vi "Drive Controller.vi"(8 "error in":errorcluster) -> ()   [LabVIEW 2019]
doc: "This VI executes continuously carrying out the current operation and responding to updates or new operation requests. It will often contain the timing or control code that is difficult to place directly in TeleOp. This VI generally opens all sensors and motors and isolates the rest of the robot code from knowing implementation details of how the operations are carried out."
uses:
  <vilib>/Rock Robotics/WPI/Framework/Completion Status.ctl
  Drive Setpoints.ctl
  Drive Operations.ctl
  <vilib>/Rock Robotics/SystemInterfaces/DIO/FPGA_DIOPWMChannel.ctl
  <vilib>/Rock Robotics/WPI/MotorControl/WPI_MotorControlOpen SPARK.vi
panel:
  in  "Interactive Values":T1
  in  "Buttons":cluster{"Execute Cmd":bool, "Abort Cmd":bool}
  out "Command Timing":cluster{"Start Time (ms)":u32, "Iterations":i32}
  out "Status":T3
  out "Setpoints":T4(graph)
  out "Current\nCmd":string
  # "Tip: The graph shows the motor setpoints. It may also be helpful to observe inputs and sensor values.\nYou may also want to display tuning or debugging controls."
  # "Interactive Command: You may fill in the settings for a command\nand schedule it with the Execute button. You can observe and abort\nany command while fine tuning the code for the controller."
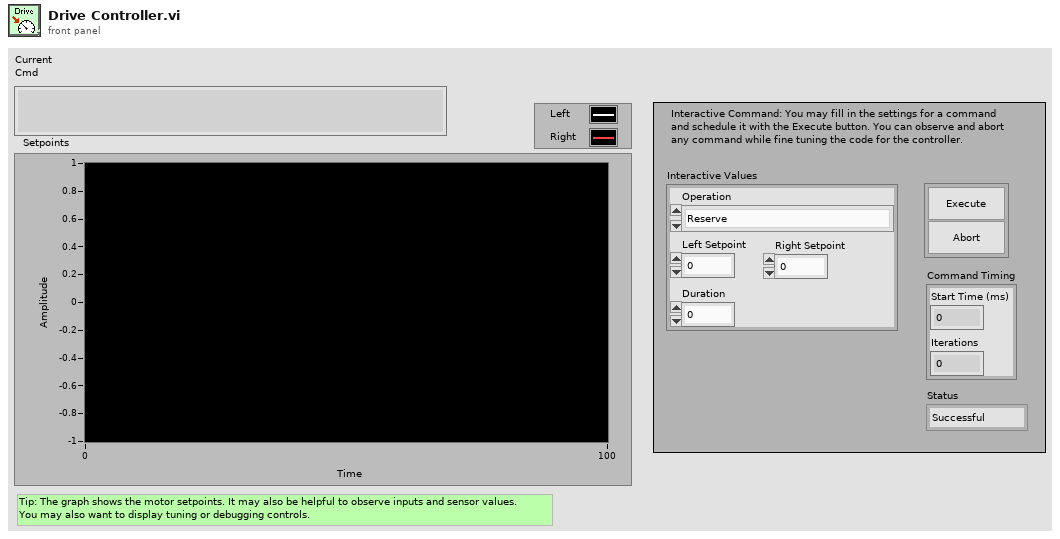
[diagram p1: front panel]
types:
  T1 = typedef "Drive Setpoints.ctl" = cluster{"Operation":T2, "Left Setpoint":dbl, "Right Setpoint":dbl, "Duration":dbl}
  T2 = typedef "Drive Operations.ctl" = enum16{"Reserve", "Read Current", "Immediate", "Drive for Time", "Drive for Distance"}
  T3 = typedef "Completion Status.ctl" = enum16{"Successful", "Aborted", "Incomplete"}
  T4 = cluster{"Left Setpoint":dbl, "Right Setpoint":dbl}
  T5 = typedef "FPGA_DIOPWMChannel.ctl" = enum8{"PWM 0", "PWM 1", "PWM 2", "PWM 3", "PWM 4", "PWM 5", "PWM 6", "PWM 7", "PWM 8", "PWM 9", "PWM MXP 0", "PWM MXP 1", "PWM MXP 2", "PWM MXP 3", "PWM MXP 4", "PWM MXP 5", "PWM MXP 6", "PWM MXP 7", "PWM MXP 8", "PWM MXP 9", "Invalid"}
  T6 = typedef "WPI_MotorControlDeviceRef.ctl" = cluster{"DeviceStatus":errorcluster, "Type":T7, "PWM":cluster{"PWM Channel":T5, "DeadBand":T8}, "CAN":cluster{"Device Number":u8, "SetOutput VI Ref":variant, "GetOutput VI Ref":variant, "Enable VI Ref":variant, "Disable VI Ref":variant, "Data":variant}, "Invert":bool, "DIO PWM":cluster{"PWM \"Enable\" Channel":T5, "DIOChannel":T9, "PWM Rate":dbl}}
  T7 = typedef "WPI_MotorControlType.ctl" = enum16{"PWM", "CAN", "DIO PWM"}
  T8 = typedef "WPI_PWMDeadband.ctl" = cluster{"Name":string, "maxPositivePwm":i32, "minPositivePwm":i32, "centerPwm":i32, "maxNegativePwm":i32, "minNegativePwm":i32, "angularRange":u16}
  T9 = typedef "FPGA_DIOChannel.ctl" = enum8{"DIO 0", "DIO 1", "DIO 2", "DIO 3", "DIO 4", "DIO 5", "DIO 6", "DIO 7", "DIO 8", "DIO 9", "DIO MXP 0", "DIO MXP 1", "DIO MXP 2", "DIO MXP 3", "DIO MXP 4", "DIO MXP 5", "DIO MXP 6", "DIO MXP 7", "DIO MXP 8", "DIO MXP 9", "DIO MXP 10", "DIO MXP 11", "DIO MXP 12", "DIO MXP 13", "DIO MXP 14", "DIO MXP 15", "SPI Port CS1", "SPI Port CS2", "SPI Port CS3", "SPI Port MISO", "SPI Port MOSI", "Invalid"}
  T10 = cluster{"MotorControlDeviceRef":T6, "MotorControlDeviceRef":T6, "MotorControlDeviceRef":T6, "MotorControlDeviceRef":T6, "error out":errorcluster, "error out":errorcluster, "error out":errorcluster, "error out":errorcluster, "MotorControlDeviceRef":T6, "error out":errorcluster, "MotorControlDeviceRef":T6, "error out":errorcluster}
  T11 = typedef "Command Status Info.ctl" = cluster{"Name":string, "Status":T3, "notifier out":T12}
  T12 = typedef "Completion Notifier.ctl" = refnum<notifier>
  T13 = cluster{"SubSystem Data":T1, cluster{"Start Time (ms)":u32, "Iterations":i32}, cluster{"Command Info":T11, "Description":string, "Default Command":T1, "queue out":refnum<queue>, "Subsystem Name":string}}
  T14 = cluster{"SubSystem Data":T1, cluster{"Start Time (ms)":u32, "Iterations":i32}, "Default Command Arguments":cluster{"Command Info":T11, "Description":string, "Default Command":T1, "queue out":refnum<queue>, "Subsystem Name":string}}
  T15 = cluster{"Don't move motors while reserved":dbl, "Don't move motors while reserved":dbl}
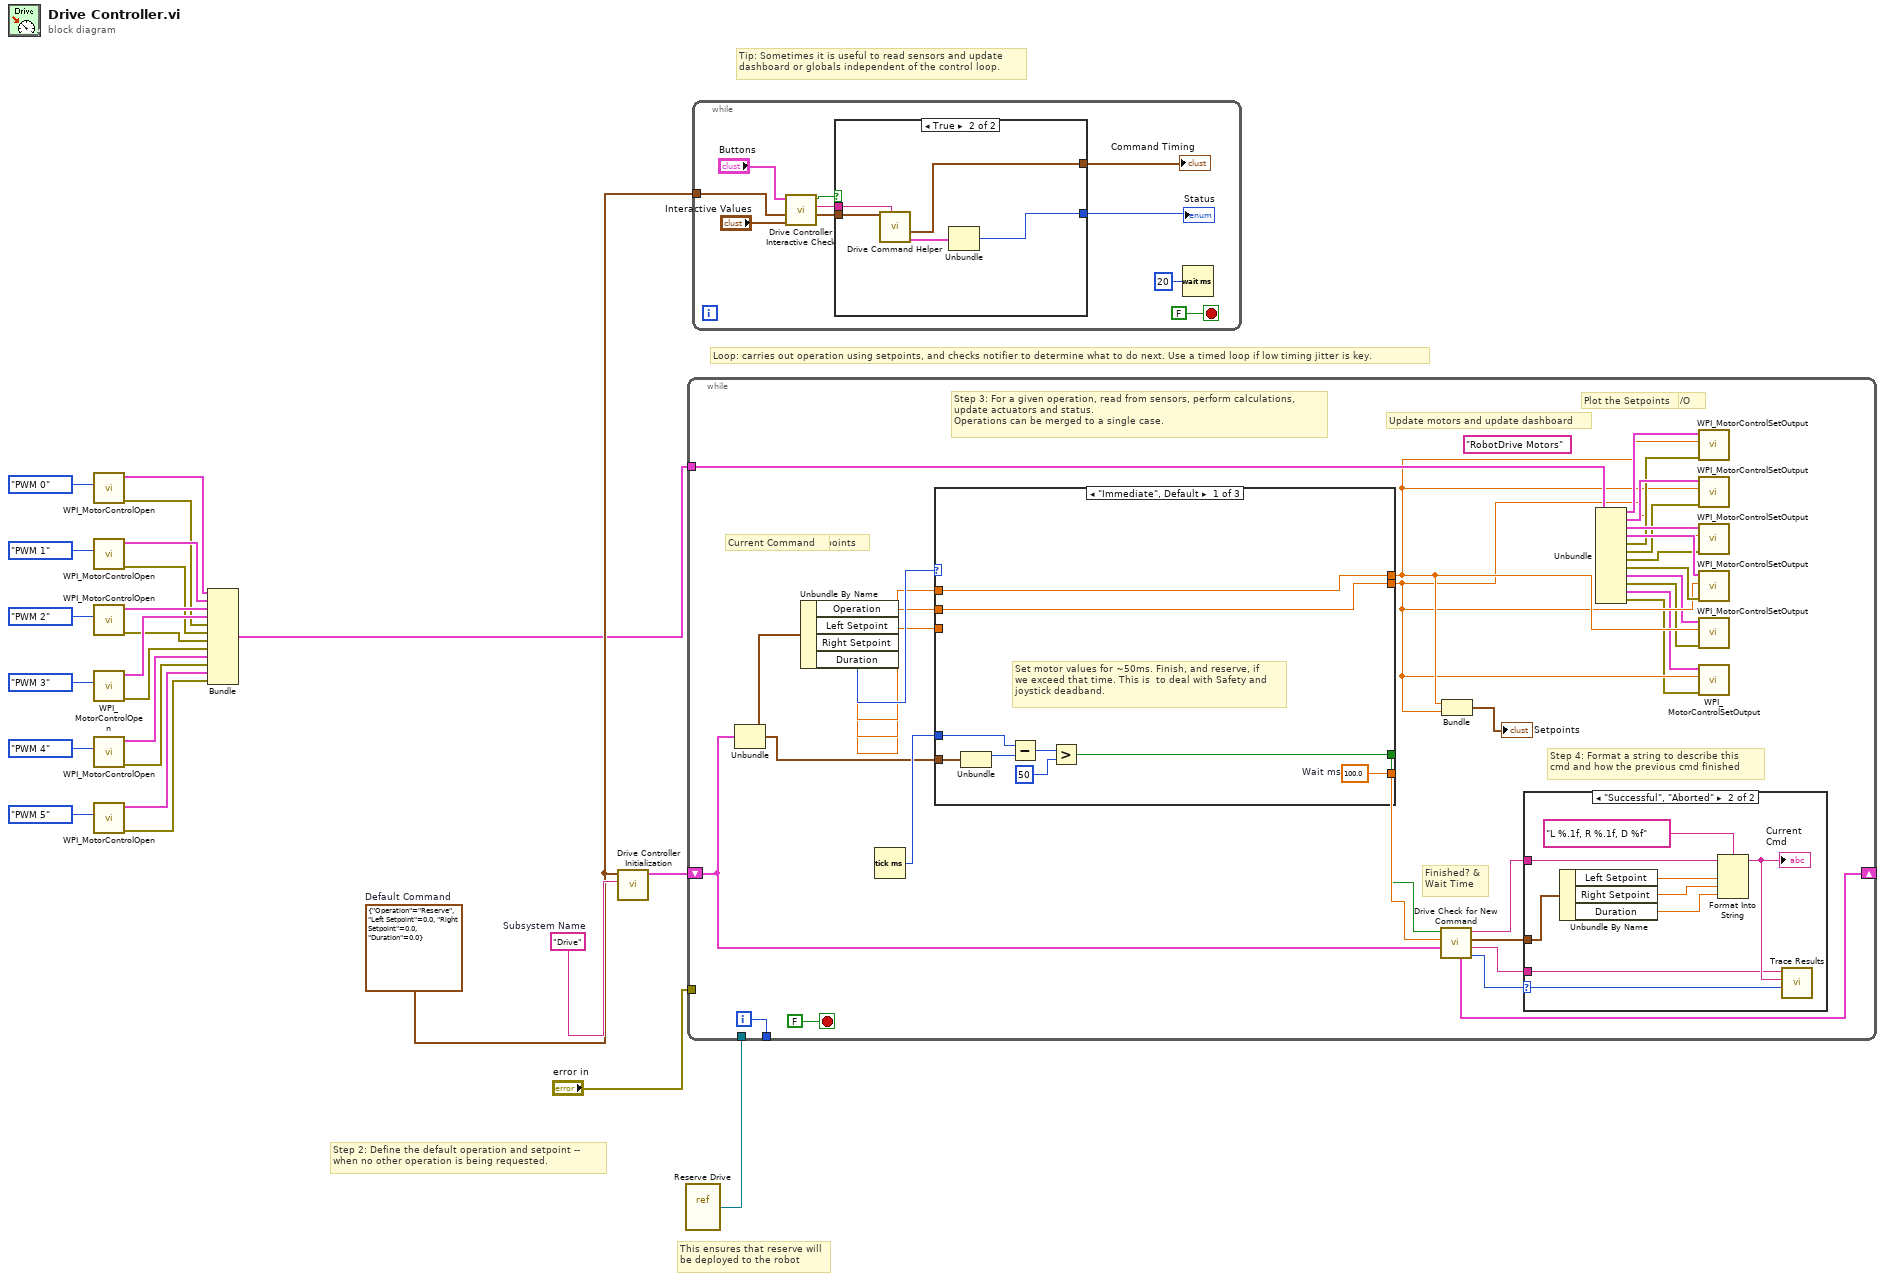
[diagram p0: block diagram]
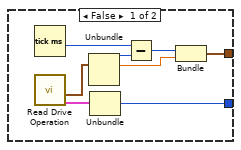
[diagram p2: hidden frame]
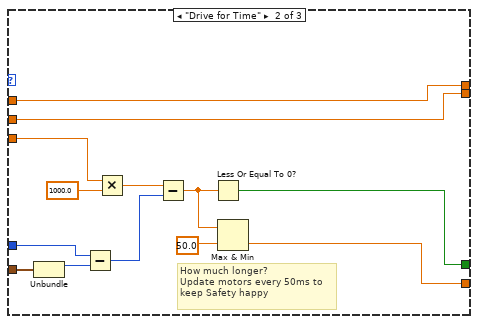
[diagram p4: hidden frame]
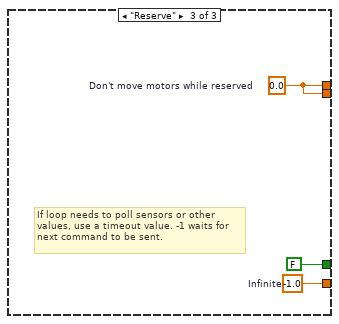
[diagram p5: hidden frame]
diagram:
  w20 = T1 {"Operation"=enum."Reserve", "Left Setpoint"=0.0, "Right Setpoint"=0.0, "Duration"=0.0}  # Default Command
  w24 = "Drive"  # Subsystem Name
  # "This ensures that reserve will\nbe deployed to the robot"
  # "Tip: Sometimes it is useful to read sensors and update\ndashboard or globals independent of the control loop."
  # "Step 2: Define the default operation and setpoint --\nwhen no other operation is being requested."
  # "Loop: carries out operation using setpoints, and checks notifier to determine what to do next. Use a timed loop if low timing jitter is key."
  n1 = call-poly <vilib>:"WPI_MotorControlOpen.vi"("PWM Channel"=FPGA_DIOPWMChannel."PWM 0") -> ("error out"=w11:errorcluster, "MotorControlDeviceRef"=w15:T6)  [unwired: 9 in]
  n2 = call-poly <vilib>:"WPI_MotorControlOpen.vi"("PWM Channel"=FPGA_DIOPWMChannel."PWM 1") -> ("error out"=w10:errorcluster, "MotorControlDeviceRef"=w14:T6)  [unwired: 9 in]
  n3 = call-poly <vilib>:"WPI_MotorControlOpen.vi"("PWM Channel"=FPGA_DIOPWMChannel."PWM 2") -> ("error out"=w9:errorcluster, "MotorControlDeviceRef"=w13:T6)  [unwired: 9 in]
  n4 = call-poly <vilib>:"WPI_MotorControlOpen.vi"("PWM Channel"=FPGA_DIOPWMChannel."PWM 3") -> ("error out"=w8:errorcluster, "MotorControlDeviceRef"=w12:T6)  [unwired: 9 in]
  n5 = call-poly <vilib>:"WPI_MotorControlOpen.vi"("PWM Channel"=FPGA_DIOPWMChannel."PWM 4") -> ("error out"=w3:errorcluster, "MotorControlDeviceRef"=w4:T6)  [unwired: 9 in]
  n6 = call-poly <vilib>:"WPI_MotorControlOpen.vi"("PWM Channel"=FPGA_DIOPWMChannel."PWM 5") -> ("error out"=w1:errorcluster, "MotorControlDeviceRef"=w2:T6)  [unwired: 9 in]
  n7 = Bundle("MotorControlDeviceRef"=w15, "MotorControlDeviceRef"=w14, "MotorControlDeviceRef"=w13, "MotorControlDeviceRef"=w12, "error out"=w11, "error out"=w10, "error out"=w9, "error out"=w8, "MotorControlDeviceRef"=w4, "error out"=w3, "MotorControlDeviceRef"=w2, "error out"=w1) -> (w7:T10)  [unwired: 1 in]
  n8 = call "Drive Controller Initialization.vi"("Subsystem Name"=w24, "Default Command"=w20) -> ("Current Command"=w22:T13)  [unwired: 9 in]
  n9 = vi-ref "Reserve Drive.vi"() -> (w21:refnum<vi>)
  n10 = while {
    shift-right: [w47] -> _
    shift-left: w22 -> [w40]
    tunnel: [w56] -> _
    tunnel: "error in" -> [_]
    tunnel: w21 -> [_]
    tunnel: w7 -> [w39]
    i -> [w56]
    stop <- FALSE stop-if-true
    (unwired) "RobotDrive Motors" ("Name")
    # "Step 5: Upate your I/O"
    # "Step 4: Format a string to describe this\ncmd and how the previous cmd finished"
    # "Current Command"
    # "Update motors and update dashboard"
    # "Plot the Setpoints"
    # "Access Cmd setpoints"
    # "Finished? &\nWait Time"
    # "Step 3: For a given operation, read from sensors, perform calculations,\nupdate actuators and status.\nOperations can be merged to a single case."
    n11 = Unbundle(w40) -> ("SubSystem Data"=w54:T1, w41:cluster{"Start Time (ms)":u32, "Iterations":i32})  [unwired: 1 out]
    n12 = Unbundle By Name(w54) -> ("Operation"=w53:T2, "Left Setpoint"=w52:dbl, "Right Setpoint"=w51:dbl, "Duration"=w50:dbl)
    n13 = Tick Count (ms)() -> (millisecond timer value=w49:u32)
    n14 = case shown="\"Immediate\", Default" w53 {
      tunnel: [w75 w76 w91] -> w46
      tunnel: [w68 w83 FALSE ("ignore previous (F)")] -> w45
      tunnel: w41 -> [w67 w85 _]
      tunnel: [w74 w82 w89] -> w30
      tunnel: [w73 w81 w89] -> w29
      tunnel: w52 -> [w74 w82 _]
      tunnel: w51 -> [w73 w81 _]
      tunnel: w50 -> [_ w80 _]
      tunnel: w49 -> [w69 w79 _]
      frame "Immediate", Default {
        w75 = 100.0  # Wait ms
        # "Set motor values for ~50ms. Finish, and reserve, if\nwe exceed that time. This is  to deal with Safety and\njoystick deadband."
        n15 = Unbundle(w67) -> ("Start Time (ms)"=w70:u32)  [unwired: 1 out]
        n16 = Subtract(x=w69, y=w70) -> (x-y=w71:u32)
        n17 = Greater?(x=w71, y=u8 50 ("Left Motor")) -> (0:w68:bool)
      }
      frame "Drive for Time" {
        # "How much longer?\nUpdate motors every 50ms to\nkeep Safety happy"
        n18 = Unbundle(w85) -> ("Start Time (ms)"=w84:u32)  [unwired: 1 out]
        n19 = Subtract(x=w79, y=w84) -> (x-y=w88:u32)
        n20 = Multiply(x=w80, y=1000.0) -> (x*y=w87:dbl)
        n21 = Subtract(x=w87, y=w88) -> (x-y=w78:dbl)
        n22 = Less Or Equal To 0?(x=w78) -> (x <= 0?=w83:bool)
        n23 = Max & Min(x=w78, y=50.0) -> (min(x,y)=w76:dbl)  [unwired: 1 out]
      }
      frame "Reserve" {
        w89 = 0.0  # Don't move motors while reserved
        w91 = -1.0  # Infinite
        # "If loop needs to poll sensors or other\nvalues, use a timeout value. -1 waits for\nnext command to be sent."
      }
    }
    n24 = call "Drive Check for New Command.vi"("input cluster"=w40, "Wait time (ms)"=w46, "Finished?"=w45) -> ("Completion"=w48:T3, "Subsystem Name"=w42:string, "Current Command"=w43:T1, "Initial Trace String"=w44:string, "Next Command"=w47:T14)  [unwired: 4 in]
    n25 = Bundle("Don't move motors while reserved"=w30, "Don't move motors while reserved"=w29) -> (→"Setpoints":T15)  [unwired: 1 in]
    n26 = case shown="\"Successful\", \"Aborted\"" w48 {
      selector: w48 -> [_ w66]
      tunnel: w44 -> [_ w61]
      tunnel: w43 -> [_ w62]
      tunnel: w42 -> [_ w58]
      frame "Incomplete", Default {
        # "Continuing current command"
      }
      frame "Successful", "Aborted" {
        # "Report and setup for next command"
        n27 = Unbundle By Name(w62) -> ("Left Setpoint"=w64:dbl, "Right Setpoint"=w65:dbl, "Duration"=w59:dbl)
        n28 = Format Into String(format string="L %.1f, R %.1f, D %f", initial string=w61, w64, w65, w59) -> (resulting string=w60:string)  [unwired: 1 in, 1 out]
        "Current\nCmd" <- w60
        n29 = call <vilib>:"Trace Results.vi"("Status of previous command"=w66, "Description"=w60, "Subsystem"=w58) -> ()  [unwired: 9 in]
      }
    }
    n30 = Unbundle(w39) -> ("MotorControlDeviceRef"=w38:T6, "MotorControlDeviceRef"=w37:T6, "MotorControlDeviceRef"=w36:T6, "MotorControlDeviceRef"=w35:T6, "error out"=w34:errorcluster, "error out"=w33:errorcluster, "error out"=w32:errorcluster, "error out"=w31:errorcluster, "MotorControlDeviceRef"=w28:T6, "error out"=w27:errorcluster, "MotorControlDeviceRef"=w26:T6, "error out"=w25:errorcluster)
    n31 = call <vilib>:"WPI_MotorControlSetOutput.vi"("error in (no error)"=w34, "Output"=w30, "MotorControlDevRef"=w38) -> ()  [unwired: 6 in, 3 out]
    n32 = call <vilib>:"WPI_MotorControlSetOutput.vi"("error in (no error)"=w33, "Output"=w30, "MotorControlDevRef"=w37) -> ()  [unwired: 6 in, 3 out]
    n33 = call <vilib>:"WPI_MotorControlSetOutput.vi"("error in (no error)"=w32, "Output"=w29, "MotorControlDevRef"=w36) -> ()  [unwired: 6 in, 3 out]
    n34 = call <vilib>:"WPI_MotorControlSetOutput.vi"("error in (no error)"=w31, "Output"=w29, "MotorControlDevRef"=w35) -> ()  [unwired: 6 in, 3 out]
    n35 = call <vilib>:"WPI_MotorControlSetOutput.vi"("error in (no error)"=w27, "Output"=w30, "MotorControlDevRef"=w28) -> ()  [unwired: 6 in, 3 out]
    n36 = call <vilib>:"WPI_MotorControlSetOutput.vi"("error in (no error)"=w25, "Output"=w29, "MotorControlDevRef"=w26) -> ()  [unwired: 6 in, 3 out]
  }
  n37 = while {
    tunnel: w20 -> [w93]
    stop <- FALSE stop-if-true
    n38 = call "Drive Controller Interactive Check.vi"("Interactive Command In"="Interactive Values", "Default Command"=w93, "Buttons"="Buttons") -> ("Interactive Command Out"=w95:T1, "Trace String"=w96:string, "Schedule"=w97:bool)  [unwired: 6 in]
    n39 = case shown="True" w97 {
      tunnel: [w106 w114] -> w98
      tunnel: [w105 w110] -> w99
      tunnel: w96 -> [_ w112]
      tunnel: w95 -> [_ w111]
      frame False {
        n40 = Tick Count (ms)() -> (millisecond timer value=w109:u32)
        n41 = call "Read Drive Operation.vi"() -> ("Command Info"=w103:T11, "SubSystem Data"=w102:T1)  [unwired: 9 in, 1 out]
        n42 = Unbundle(w102) -> ("Operation"=w107:T2, "Left Setpoint"=w104:dbl)  [unwired: 2 out]
        n43 = Unbundle(w103) -> ("Status"=w106:T3)  [unwired: 2 out]
        n44 = Subtract(x=w109, y=w107) -> (x-y=w108:u32)
        n45 = Bundle(w108, "Left Setpoint"=w104) -> (w105:cluster{u32, "Left Setpoint":dbl})  [unwired: 1 in]
      }
      frame True {
        n46 = call "Drive Command Helper.vi"("Description"=w112, "SubSystem Data"=w111) -> ("Command Info Out"=w113:T11, "Command Timing"=w110:cluster{"Start Time (ms)":u32, "Iterations":i32})  [unwired: 7 in, 1 out]
        n47 = Unbundle(w113) -> ("Status"=w114:T3)  [unwired: 2 out]
      }
    }
    "Status" <- w98
    "Command Timing" <- w99
    n48 = Wait (ms)(milliseconds to wait=u32 20) -> ()  [unwired: 1 out]
  }
